vi "ForceTunnel.vi"(5 "curret PelvicP":dbl[](array[numeric])) -> (1 "ForceXYZ":dbl[](array[numeric]))   [LabVIEW 2013]
uses:
  ForceField/TypeDef/FTconst.ctl
  ForceField/TypeDef/AnkleTrajPt.ctl
  <vilib>/Analysis/baseanly.llb/Real Dot Product.vi
  <vilib>/Analysis/_algsub.llb/Real Vector Norm.vi
  <vilib>/Analysis/BLAS.llb/idamin - Min Element Index (DBL).vi
  <vilib>/Analysis/NI_AALBase.lvlib
  <vilib>/Analysis/NI_AALPro.lvlib
  <vilib>/Analysis/NI_AALBLAS.lvlib
  ForceField/ForceField.lvclass
panel:
  out "appended array 2":dbl[](array[numeric])
  out "ActiveTraj":dbl[][](array[numeric])
  in  "HalfWindow":i32=60
  in  "Init":bool
  out "Closest Pt":dbl[](array[numeric])
  out "d_min":dbl
  out "n_dir":dbl[](array[numeric])
  in  "Enum":enum16{"Linear", "Bell"}(ring)
  in  "FT Constant":T1
  out "ForceComp":dbl[](array[numeric])
  out "TangentVectorAtClosestPt":dbl[](array[numeric])
  out "NormalVectorToClosestPt":dbl[](array[numeric])
  out "DistanceToClosestPt":dbl
  out "IndexOfClosePt":i32
  out "Array 2":dbl[][](array[numeric])
  in  "stop":bool
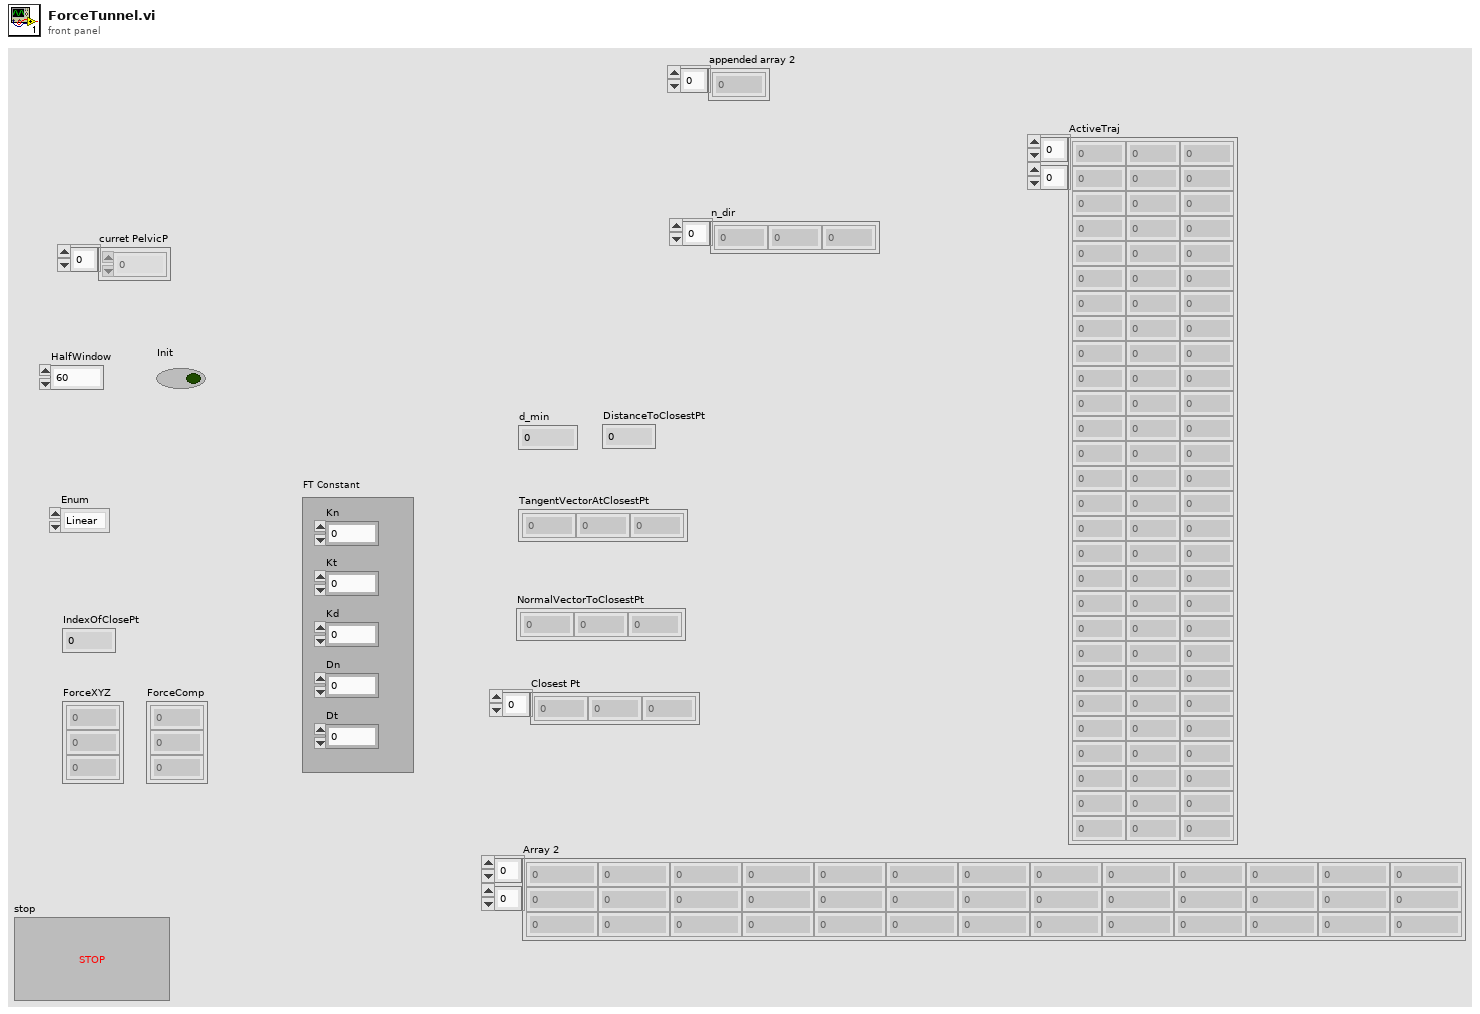
[diagram p1: front panel]
types:
  T1 = typedef "FTconst.ctl" = cluster{"Kn":dbl, "Kt":dbl, "Kd":dbl, "Dn":dbl, "Dt":dbl}
  T2 = typedef "ForceField.lvclass/AnkleTrajPt.ctl" = cluster{"P1":dbl[], "P2":dbl[], "P1-P2":dbl[], "(P1-P2)^2":dbl}
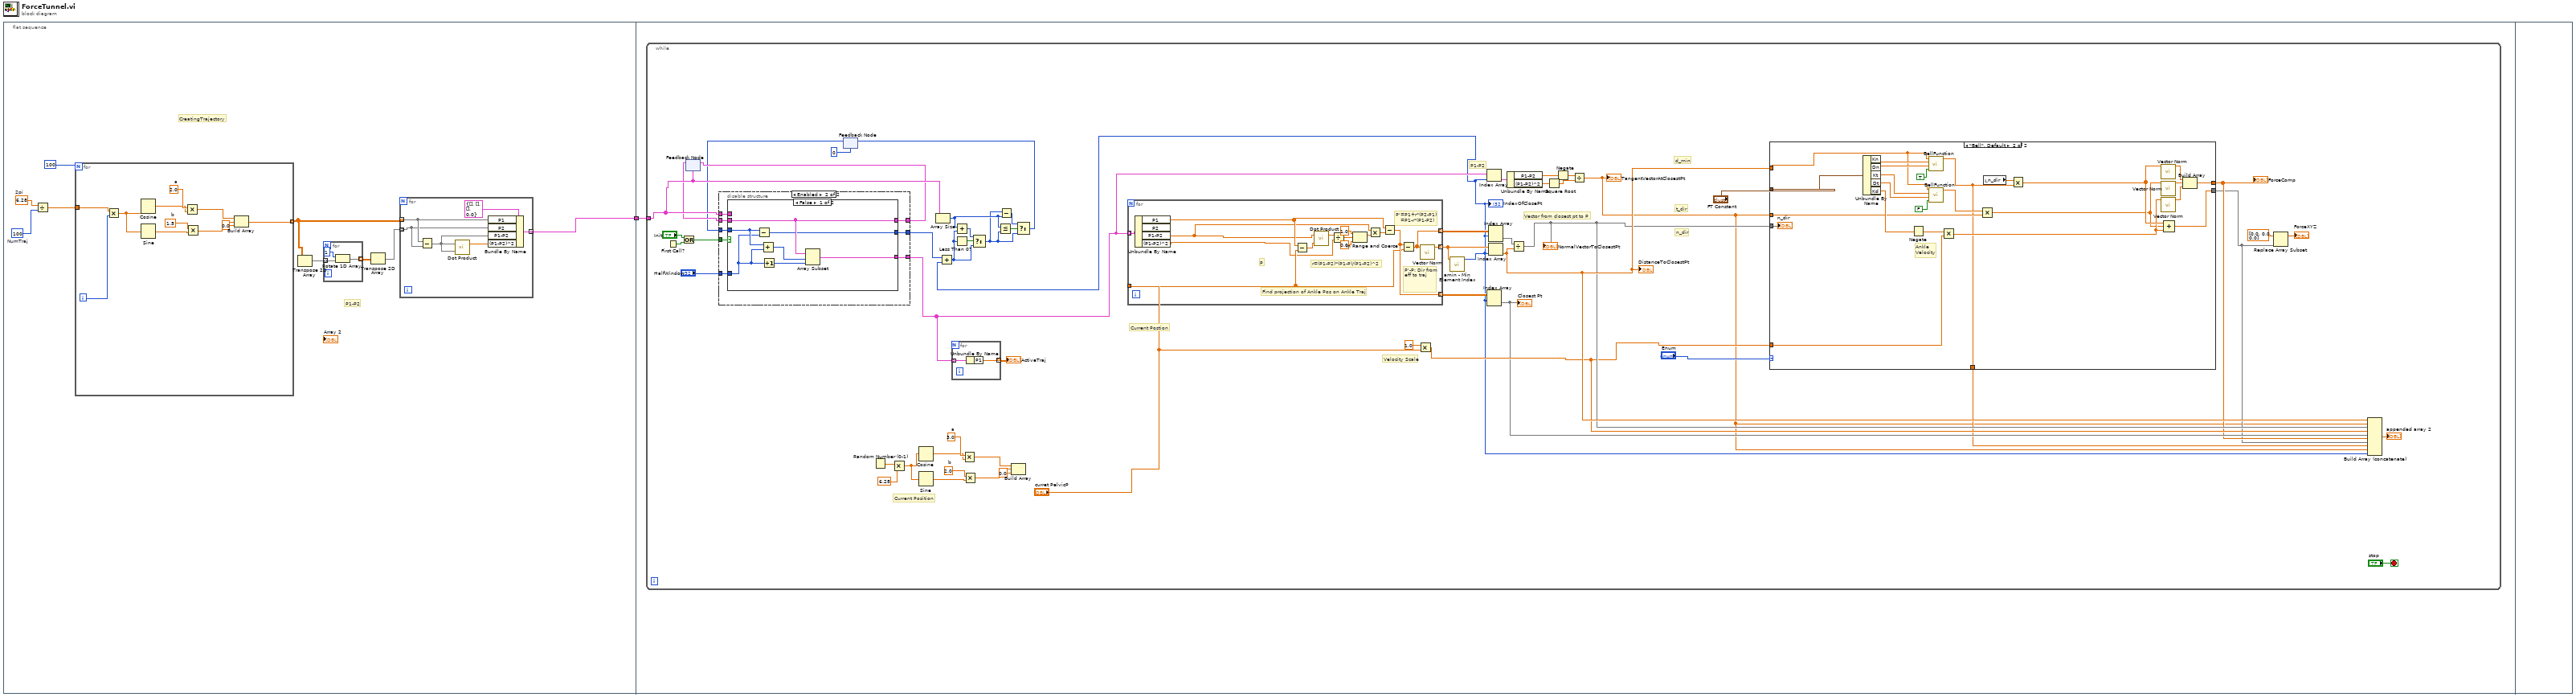
[diagram p0: block diagram]
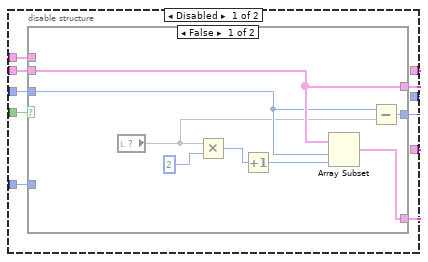
[diagram p2: hidden frame]
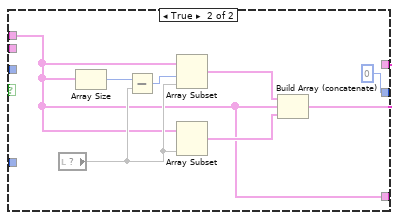
[diagram p3: hidden frame]
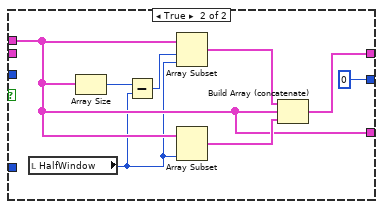
[diagram p4: hidden frame]
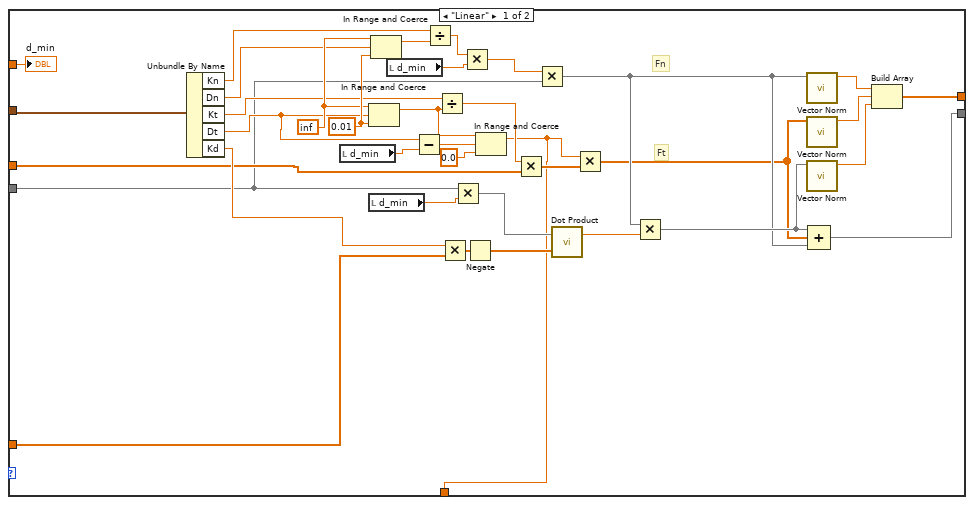
[diagram p5: hidden frame]
diagram:
  n1 = flat-sequence {
    tunnel: [w3] -> w1
    tunnel: w1 -> [w31]
    frame #0 {
      w6 = 6.28  # 2pi
      w7 = 100  # NumTraj
      # "CreatingTrajectory"
      # "P1-P2"
      n2 = Divide(x=w6, y=w7) -> (x/y=w8:dbl)
      n3 = for {
        N: 100 -> [_]
        tunnel: w8 -> [w27]
        tunnel: [w19] -> w4 mode=indexing
        i -> [w26]
        w23 = 1.5  # b
        w25 = 2.0  # a
        n4 = Multiply(x=w27, y=w26) -> (x*y=w24:dbl)
        n5 = Cosine(x=w24) -> (cos(x)=w18:dbl)
        n6 = Sine(x=w24) -> (sin(x)=w17:dbl)
        n7 = Multiply(x=w25, y=w18) -> (x*y=w22:dbl)
        n8 = Multiply(x=w23, y=w17) -> (x*y=w21:dbl)
        n9 = Build Array(w22, w21, 0.0 ("element")) -> (w19:dbl[])
      }
      n10 = Transpose 2D Array(2D array=w4) -> (transposed array=w5:dbl[][])
      n11 = for {
        tunnel: w5 -> [w30] mode=indexing
        tunnel: [w28] -> w10 mode=indexing
        n12 = Rotate 1D Array(1:w30, 2:1 ("n")) -> (0:w28:dbl[])
      }
      n13 = Transpose 2D Array(2D array=w10) -> (transposed array=w2:dbl[][])
      n14 = for {
        tunnel: w4 -> [w15] mode=indexing
        tunnel: [w16] -> w3 mode=indexing
        tunnel: w2 -> [w11] mode=indexing
        n15 = Subtract(x=w15, y=w11) -> (x-y=w13:dbl[])
        n16 = call-poly <vilib>:"Dot Product.vi"("Y Vector"=w13, "X Vector"=w13) -> ("X * Y"=w12:dbl)  [unwired: 1 out]
        n17 = Bundle By Name(cluster=T2 {"P1"=[], "P2"=[], "P1-P2"=[], "(P1-P2)^2"=0.0} ("AnkleTraj"), "P1"=w15, "P2"=w11, "P1-P2"=w13, "(P1-P2)^2"=w12) -> (w16:T2)
      }
    }
    frame #1 {
      n18 = while {
        tunnel: w31 -> [w43]
        stop <- "stop" stop-if-true
        w77 = 2.0  # b
        w78 = 3.0  # a
        # "Current Postion"
        # "Velocity Scale"
        # "Current Position"
        # "P1-P2"
        # "t_dir"
        # "n_dir"
        # "d_min"
        # "Vector from closest pt to P"
        n19 = First Call?() -> (First Call?: T/F=w45:bool)
        n20 = Or(x="Init", y=w45) -> (x .or. y?=w42:bool)
        n21 = feedback #1(w43) -> (w40:T2[])
        n22 = feedback #2(0) -> (w37:i32)
        n23 = disable-structure shown="Enabled" {
          disable-tunnel: w42 -> [w97 w121]
          disable-tunnel: w37 -> [w96 w114]
          disable-tunnel: [w95 w120] -> w35
          disable-tunnel: w40 -> [w94 w115]
          disable-tunnel: [w93 w119] -> w38
          disable-tunnel: [w92 w118] -> w39
          disable-tunnel: w43 -> [w91 w117]
          disable-tunnel: "HalfWindow" -> [w90 w116]
          frame Disabled {
            n24 = case shown="False" w97 {
              tunnel: w96 -> [w100 _]
              tunnel: w94 -> [w104 _]
              tunnel: [w105 w106] -> w95
              tunnel: [w104 w108] -> w93
              tunnel: [w99 0] -> w92
              tunnel: w91 -> [_ w106]
              tunnel: w90 -> [_ _]
              frame False {
                n25 = local read item#-1() -> (w98)
                n26 = Multiply(x=w98, y=2) -> (x*y=w103:i32)
                n27 = Increment(x=w103) -> (x+1=w102:i32)
                n28 = Array Subset(array=w104, index=w100, length=w102) -> (w105:T2[])
                n29 = Subtract(x=w100, y=w98) -> (x-y=w99:i32)
              }
              frame True {
                n30 = local read item#-1() -> (w112)
                n31 = Array Size(array=w106) -> (size(s)=w113:i32)
                n32 = Subtract(x=w113, y=w112) -> (x-y=w111:i32)
                n33 = Array Subset(array=w106, index=w111, length=w112) -> (w109:T2[])
                n34 = Array Subset(array=w106, length=w112) -> (w110:T2[])  [unwired: 1 in]
                n35 = Build Array (concatenate)(w109, w106, w110) -> (w108:T2[])
              }
            }
          }
          frame Enabled {
            n36 = case shown="False" w121 {
              tunnel: w114 -> [w125 _]
              tunnel: w115 -> [w128 _]
              tunnel: [w122 w130] -> w120
              tunnel: [w128 w132] -> w119
              tunnel: [w126 0] -> w118
              tunnel: w117 -> [_ w130]
              tunnel: w116 -> [w124 _]
              frame False {
                n37 = Subtract(x=w125, y=w124) -> (x-y=w126:i32)
                n38 = Add(x=w125, y=w124) -> (x+y=w123:i32)
                n39 = Increment(x=w124) -> (x+1=w127:i32)
                n40 = Array Subset(array=w128, index=w123, length=w127) -> (w122:T2[])
              }
              frame True {
                n41 = local read "HalfWindow"() -> (w129:i32)
                n42 = Array Size(array=w130) -> (size(s)=w136:i32)
                n43 = Subtract(x=w136, y=w129) -> (x-y=w135:i32)
                n44 = Array Subset(array=w130, index=w135, length=w129) -> (w133:T2[])
                n45 = Array Subset(array=w130, length=w129) -> (w134:T2[])  [unwired: 1 in]
                n46 = Build Array (concatenate)(w133, w130, w134) -> (w132:T2[])
              }
            }
          }
        }
        n47 = feedback-in #1(w38) -> ()
        n48 = Random Number (0-1)() -> (number: 0 to 1=w71:dbl)
        n49 = Multiply(x=w71, y=6.28) -> (x*y=w70:dbl)
        n50 = Cosine(x=w70) -> (cos(x)=w73:dbl)
        n51 = Sine(x=w70) -> (sin(x)=w72:dbl)
        n52 = Array Size(array=w43) -> (size(s)=w48:i32)
        n53 = for {
          tunnel: w35 -> [w89] mode=indexing
          tunnel: [w88] -> w36 mode=indexing
          n54 = Unbundle By Name(w89) -> ("P1"=w88:dbl[])
        }
        "ActiveTraj" <- w36
        n55 = Multiply(x=w78, y=w73) -> (x*y=w76:dbl)
        n56 = Multiply(x=w77, y=w72) -> (x*y=w75:dbl)
        n57 = Build Array(w76, w75, 0.0 ("element")) -> ()  [unwired: 1 out]
        n58 = for {
          tunnel: [w204] -> w83 mode=indexing
          tunnel: [w203] -> w84 mode=indexing
          tunnel: [w202] -> w86 mode=indexing
          tunnel: w35 -> [w197] mode=indexing
          tunnel: "curret PelvicP" -> [w201]
          # "P"
          # "P'-P: Dir from eff to traj"
          # "r=(P1-P2)*(P1-P)/(P1-P2)^2"
          # "P'=P1+r*(P2-P1)\n   =P1-r*(P1-P2)"
          # "Find projection of Ankle Pos on Ankle Traj"
          n59 = Unbundle By Name(w197) -> ("P1"=w200:dbl[], "P1-P2"=w199:dbl[], "(P1-P2)^2"=w198:dbl)  [unwired: 1 out]
          n60 = Subtract(x=w200, y=w201) -> (x-y=w211:dbl[])
          n61 = call-poly <vilib>:"Dot Product.vi"("Y Vector"=w211, "X Vector"=w199) -> ("X * Y"=w210:dbl)  [unwired: 1 out]
          n62 = Divide(x=w210, y=w198) -> (x/y=w209:dbl)
          n63 = In Range and Coerce(upper limit=1.0, x=w209, lower limit=0.0) -> (coerced(x)=w206:dbl)  [unwired: 1 out]
          n64 = Multiply(x=w199, y=w206) -> (x*y=w205:dbl[])
          n65 = Subtract(x=w200, y=w205) -> (x-y=w202:dbl[])
          n66 = Subtract(x=w202, y=w201) -> (x-y=w203:dbl[])
          n67 = call-poly <vilib>:"Vector Norm.vi"("Input Vector"=w203) -> ("norm"=w204:dbl)  [unwired: 9 in, 1 out]
        }
        n68 = Multiply(x=1.0, y="curret PelvicP") -> (x*y=w65:dbl[])
        n69 = call-poly <vilib>:"amin - Min Element Index.vi"("x"=w83) -> ("idamin"=w34:i32)  [unwired: 9 in, 1 out]
        "IndexOfClosePt" <- w34
        n70 = Add(x=w39, y=w34) -> (x+y=w46:i32)
        n71 = Add(x=w48, y=w46) -> (x+y=w49:i32)
        n72 = Less Than 0?(x=w46) -> (x < 0?=w50:bool)
        n73 = Select(t=w49, s=w50, f=w46) -> (s? t:f=w47:i32)
        n74 = Less Or Equal?(x=w48, y=w47) -> (x <= y?=w53:bool)
        n75 = Subtract(x=w47, y=w48) -> (x-y=w51:i32)
        n76 = Select(t=w51, s=w53, f=w47) -> (s? t:f=w52:i32)
        n77 = feedback-in #2(w52) -> ()
        n78 = Index Array(array=w35, index=w34) -> (element=w56:T2)
        n79 = Index Array(array=w86, index (row)=w34) -> (element=w64:dbl[])  [unwired: 1 in]
        "Closest Pt" <- w64
        n80 = Index Array(array=w84, index (row)=w34) -> (element=w85:dbl[])  [unwired: 1 in]
        n81 = Index Array(array=w83, index=w34) -> (element=w67:dbl)
        "DistanceToClosestPt" <- w67
        n82 = Unbundle By Name(w56) -> ("P1-P2"=w59:dbl[], "(P1-P2)^2"=w60:dbl)
        n83 = Divide(x=w85, y=w67) -> (x/y=w66:dbl[])
        "NormalVectorToClosestPt" <- w66
        n84 = Square Root(x=w60) -> (sqrt(x)=w58:dbl)
        n85 = Negate(x=w59) -> (-x=w57:dbl[])
        n86 = Divide(x=w57, y=w58) -> (x/y=w55:dbl[])
        "TangentVectorAtClosestPt" <- w55
        n87 = case shown="\"Bell\", Default" "Enum" {
          tunnel: [w172 w189] -> w63
          tunnel: [w151 w196] -> w62
          tunnel: w65 -> [w171 w193]
          tunnel: "FT Constant" -> [w150 w187]
          tunnel: w55 -> [w144 w178]
          tunnel: w67 -> [w142 w175]
          tunnel: w66 -> [w143 w177]
          tunnel: [w137 w173] -> w61
          frame "Linear" {
            w156 = inf
            w157 = 0.01 ("upper limit")
            # "Ft"
            # "Fn"
            n88 = Unbundle By Name(w150) -> ("Kn"=w149:dbl, "Dn"=w148:dbl, "Kt"=w147:dbl, "Dt"=w146:dbl, "Kd"=w145:dbl)
            n89 = local read "d_min"() -> (w140:dbl)
            n90 = In Range and Coerce(upper limit=w156, x=w146, lower limit=w157) -> (coerced(x)=w158:dbl)  [unwired: 1 out]
            n91 = local read "d_min"() -> (w139:dbl)
            n92 = In Range and Coerce(upper limit=w156, x=w148, lower limit=w157) -> (coerced(x)=w159:dbl)  [unwired: 1 out]
            n93 = local read "d_min"() -> (w141:dbl)
            n94 = Subtract(x=w146, y=w140) -> (x-y=w162:dbl)
            n95 = Divide(x=w149, y=w159) -> (x/y=w155:dbl)
            n96 = Divide(x=w147, y=w158) -> (x/y=w160:dbl)
            n97 = Multiply ("Multiply.vi")(x=w145, y=w171) -> (x*y=w167:dbl[])
            n98 = Multiply(x=w143, y=w139) -> (x*y=w166:dbl[])
            n99 = Multiply(x=w155, y=w141) -> (x*y=w154:dbl)
            n100 = Negate(x=w167) -> (-x=w165:dbl[])
            n101 = In Range and Coerce(upper limit=w158, x=w162, lower limit=0.0) -> (coerced(x)=w137:dbl)  [unwired: 1 out]
            n102 = Multiply(x=w160, y=w144) -> (x*y=w163:dbl[])
            n103 = Multiply(x=w154, y=w143) -> (x*y=w152:dbl[])
            n104 = call-poly <vilib>:"Dot Product.vi"("Y Vector"=w165, "X Vector"=w166) -> ("X * Y"=w164:dbl)  [unwired: 1 out]
            n105 = Multiply(x=w137, y=w163) -> (x*y=w138:dbl[])
            n106 = Multiply(x=w152, y=w164) -> (x*y=w153:dbl[])
            n107 = call-poly <vilib>:"Vector Norm.vi"("Input Vector"=w152) -> ("norm"=w168:dbl)  [unwired: 9 in, 1 out]
            n108 = call-poly <vilib>:"Vector Norm.vi"("Input Vector"=w138) -> ("norm"=w169:dbl)  [unwired: 9 in, 1 out]
            n109 = call-poly <vilib>:"Vector Norm.vi"("Input Vector"=w153) -> ("norm"=w170:dbl)  [unwired: 9 in, 1 out]
            n110 = Compound Arithmetic op=ADD(w153, w138, w152) -> (w151:dbl[])
            n111 = Build Array(w168, w169, w170) -> (w172:dbl[])
            "d_min" <- w142
          }
          frame "Bell", Default {
            # "Ankle\nVelocity"
            n112 = Unbundle By Name(w187) -> ("Kn"=w180:dbl, "Dn"=w181:dbl, "Kt"=w182:dbl, "Dt"=w183:dbl, "Kd"=w186:dbl)
            n113 = Negate(x=w186) -> (-x=w188:dbl)
            n114 = call "BellFunction.vi"("Invert"=TRUE, "(r)adius"=w181, "(A)mplitude"=w180, "x"=w175) -> ("y"=w173:dbl)  [unwired: 2 in]
            n115 = call "BellFunction.vi"("Invert"=FALSE, "(r)adius"=w183, "(A)mplitude"=w182, "x"=w175) -> ("y"=w179:dbl)  [unwired: 2 in]
            n116 = Multiply(x=w188, y=w193) -> (x*y=w194:dbl[])
            n117 = Multiply(x=w179, y=w178) -> (x*y=w174:dbl[])
            n118 = local read "n_dir"() -> (w176:dbl[])
            n119 = Multiply(x=w176, y=w173) -> (x*y=w195:dbl[])
            n120 = call-poly <vilib>:"Vector Norm.vi"("Input Vector"=w195) -> ("norm"=w192:dbl)  [unwired: 9 in, 1 out]
            n121 = call-poly <vilib>:"Vector Norm.vi"("Input Vector"=w174) -> ("norm"=w191:dbl)  [unwired: 9 in, 1 out]
            n122 = call-poly <vilib>:"Vector Norm.vi"("Input Vector"=w194) -> ("norm"=w190:dbl)  [unwired: 9 in, 1 out]
            n123 = Compound Arithmetic op=ADD(w195, w174, w194) -> (w196:dbl[])
            n124 = Build Array(w192, w191, w190) -> (w189:dbl[])
            "n_dir" <- w177
          }
        }
        "ForceComp" <- w63
        n125 = Replace Array Subset(array=dbl[] [0.0, 0.0, 0.0], new element=w62) -> (→"ForceXYZ":dbl[])  [unwired: 1 in]
        n126 = Build Array (concatenate)(w67, w55, w66, w65, w64, w63, w62, w61, w55, w34) -> (→"appended array 2":dbl[])
      }
    }
    frame #2 {
    }
  }
